vi "Select PA gain.vi"() -> (1 "PA gain selected":u8)   [LabVIEW 2015, in "VIPM2.lvlib"]
doc: "Obre una finestra emergent per seleccionar el PA gain = [0..3].\nDreceres de teclat: F1..4."
uses:
  VIPM2.lvlib
panel:
  in  "x4 Button":bool
  in  "x3 Button":bool
  in  "x2 Button":bool
  in  "x1 Button":bool
  # "Select the PreAmplifier gain (PA gain)"
  # "~750 keV"
  # "~1400 keV"
  # "~2900 keV"
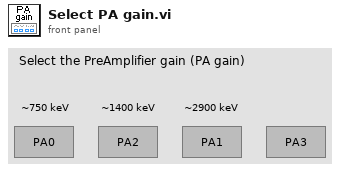
[diagram p1: front panel]
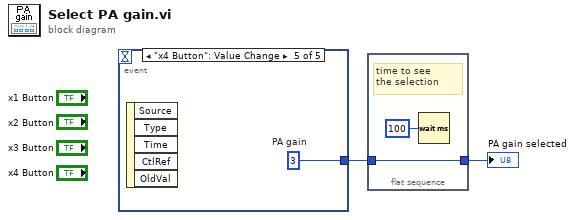
[diagram p0: block diagram]
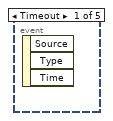
[diagram p2: hidden frame]
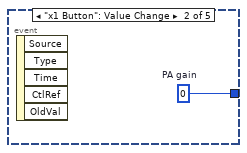
[diagram p3: hidden frame]
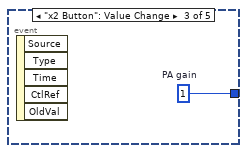
[diagram p4: hidden frame]
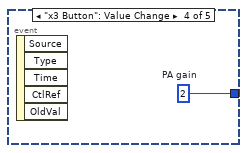
[diagram p5: hidden frame]
diagram:
  n1 = event shown="[4] \"x4 Button\": Value Change" {
    selector: _ -> [_ _ _ _ _]
    dyn-events: _ -> [_ _ _ _ _]
    timeout: _ -> [_ _ _ _ _]
    tunnel: [_ w3 w4 w5 w6] -> w1
    event Timeout {
      n2 = event-data() -> ()  [unwired: 1 in, 3 out]
    }
    event "x1 Button": Value Change {
      w3 = u8 0  # PA gain
      n3 = event-data() -> ()  [unwired: 1 in, 5 out]
    }
    event "x2 Button": Value Change {
      w4 = u8 1  # PA gain
      n4 = event-data() -> ()  [unwired: 1 in, 5 out]
    }
    event "x3 Button": Value Change {
      w5 = u8 2  # PA gain
      n5 = event-data() -> ()  [unwired: 1 in, 5 out]
    }
    event "x4 Button": Value Change {
      w6 = u8 3  # PA gain
      n6 = event-data() -> ()  [unwired: 1 in, 5 out]
    }
  }
  n7 = flat-sequence {
    tunnel: [w8] -> w2
    tunnel: w1 -> [w8]
    frame #0 {
      # "time to see\nthe selection"
      n8 = Wait (ms)(milliseconds to wait=u32 100) -> ()  [unwired: 1 out]
    }
  }
  "PA gain selected" <- w2
